vi "Read address.vi"(8 "error in (no error)":errorcluster, 11 "RemoteControl in":refnum<class "RemoteControl.lvclass">) -> (0 "error out":errorcluster, 2 "address":string, 3 "RemoteControl out":refnum<class "RemoteControl.lvclass">)   [LabVIEW 2016, in "RemoteControl.lvclass"]
uses:
  RemoteControl.lvclass
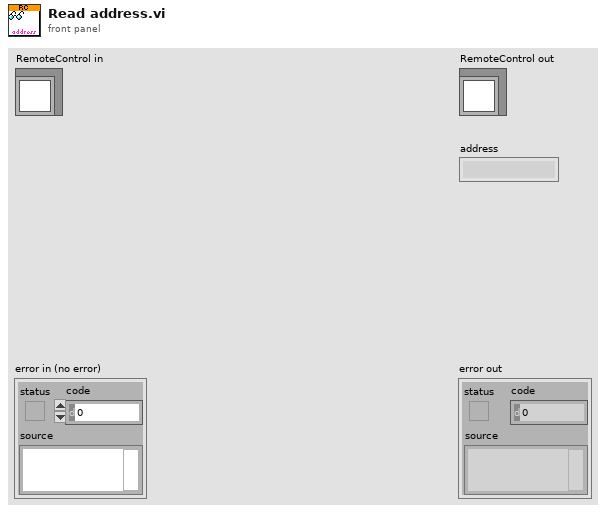
[diagram p1: front panel]
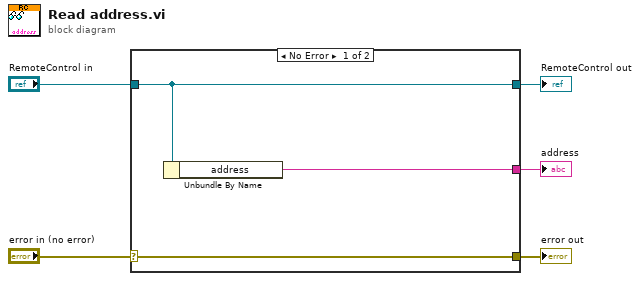
[diagram p0: block diagram]
diagram:
  n1 = case shown="No Error" "error in (no error)" {
    selector: "error in (no error)" -> [w8 w9]
    tunnel: [w8 w9] -> w4
    tunnel: [w7 w10] -> w2
    tunnel: "RemoteControl in" -> [w7 w10]
    tunnel: [w6 _] -> w1
    frame No Error {
      n2 = Unbundle By Name(w7) -> ("address"=w6:string)
    }
    frame Error {
    }
  }
  "error out" <- w4
  "RemoteControl out" <- w2
  "address" <- w1
